vi "Write Image.vi"(8 "error in (no error)":errorcluster, 9 "2D Picture":picture, 11 "64x128 I2C OLED SSD1315 In":refnum<class "64x128 I2C OLED SSD1315.lvclass">) -> (0 "error out":errorcluster, 3 "64x128 I2C OLED SSD1315 Out":refnum<class "64x128 I2C OLED SSD1315.lvclass">)   [LabVIEW 2020, in "CTI-Peripheral.lvlib" / "64x128 I2C OLED SSD1315.lvclass"]
uses:
  64x128 I2C OLED SSD1315/64x128 I2C OLED SSD1315.lvclass
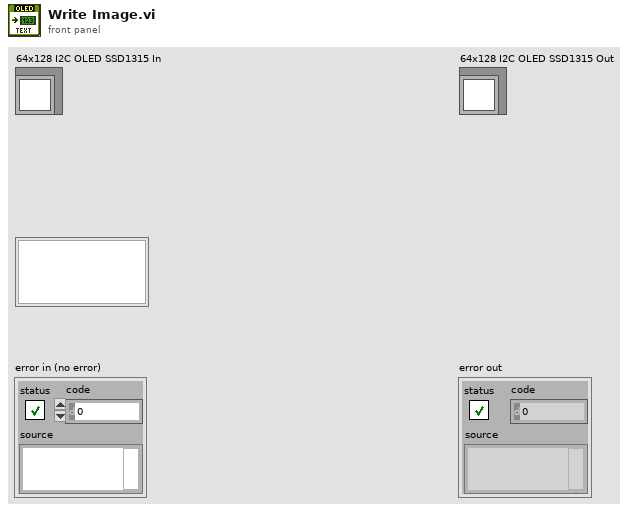
[diagram p1: front panel]
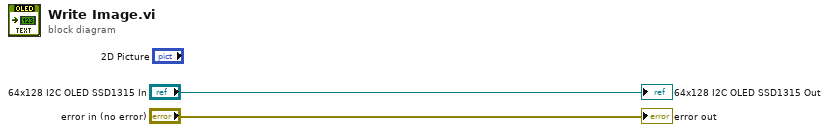
[diagram p0: block diagram]
diagram:
  "error out" <- "error in (no error)"
  "64x128 I2C OLED SSD1315 Out" <- "64x128 I2C OLED SSD1315 In"
